vi "Reset Subsystem Overviews.vi"(8 "error in (no error)":errorcluster, 11 "Subsystem Controls In":refnum<vi>[](array[refnum])) -> (0 "error out":errorcluster, 3 "Subsystem Controls Out":refnum<vi>[](array[refnum]))   [LabVIEW 2024]
doc: "Resets the subsystem overview controls."
uses:
  Controls/Client/Subsystem Overview.ctl
  Controls/Client/Alarm LED.ctl
  Controls/Client/Status LED.ctl
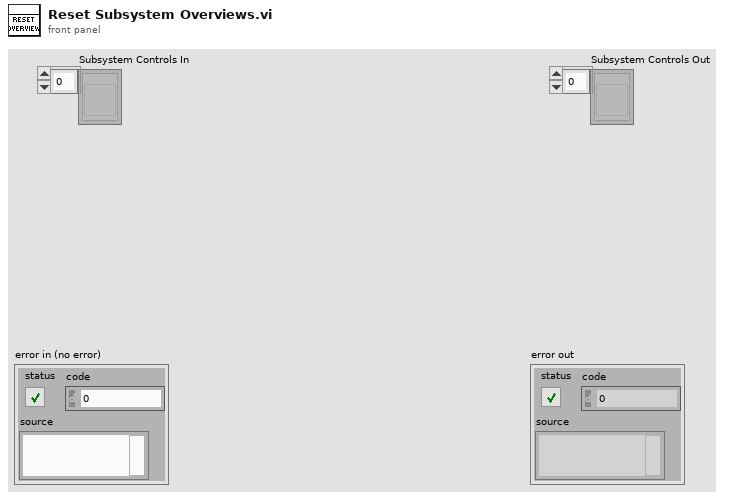
[diagram p1: front panel]
types:
  T1 = enum8{"Enabled", "Disabled", "Disabled and Grayed Out"}
  T2 = typedef "Subsystem Overview.ctl" = cluster{"Subsystem Name":string, "Description":string, "p":dbl, "i":dbl, "d":dbl, "PV":dbl, "SP":dbl, "dt":dbl, "output":dbl, "Alarming?":T3, "In use?":T4}
  T3 = typedef "Alarm LED.ctl" = bool
  T4 = typedef "Status LED.ctl" = bool
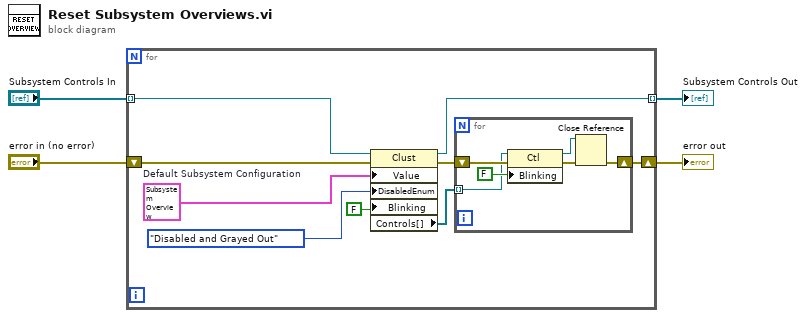
[diagram p0: block diagram]
diagram:
  n1 = for {
    tunnel: "Subsystem Controls In" -> [w11] mode=indexing
    tunnel: [w10] -> w2 mode=indexing
    shift-right: [w8] -> w1
    shift-left: "error in (no error)" -> [w12]
    w13 = T2 {"Subsystem Name"="", "Description"="", "p"=0.0, "i"=0.0, "d"=0.0, "PV"=0.0, "SP"=0.0, "dt"=0.0, "output"=0.0, "Alarming?"=FALSE, "In use?"=FALSE}  # Default Subsystem Configuration
    n2 = property class="Clust"(reference=w11, error in=w12, "Value"=w13, "DisabledEnum"=T1."Disabled and Grayed Out" ("Disabled"), "Blinking"=FALSE) -> (reference out=w10:refnum<vi>, error out=w9:errorcluster, "Controls[]"=w7:refnum<vi>[])
    n3 = for {
      shift-right: [w17] -> w8
      shift-left: w9 -> [w16]
      tunnel: w7 -> [w14] mode=indexing
      n4 = property class="Ctl"(reference=w14, error in=w16, "Blinking"=FALSE) -> (reference out=w19:refnum<vi>, error out=w18:errorcluster)
      n5 = Close Reference(reference=w19, error in (no error)=w18) -> (error out=w17:errorcluster)
    }
  }
  "error out" <- w1
  "Subsystem Controls Out" <- w2
